vi "Close.vi"(8 "error in (no error)":errorcluster, 11 "Data.TDMS in":refnum<class "Data.PG.lvclass">) -> (0 "error out":errorcluster, 3 "Data.TDMS out":refnum<class "Data.PG.lvclass">)   [LabVIEW 2020, in "Data.PG.lvclass"]
uses:
  Data.PG.lvclass
  <vilib>/JDP Science/PostgreSQL Library/Connection/PQ Connection.lvclass
  Data.PG.lvclass/Data.PG.ctl
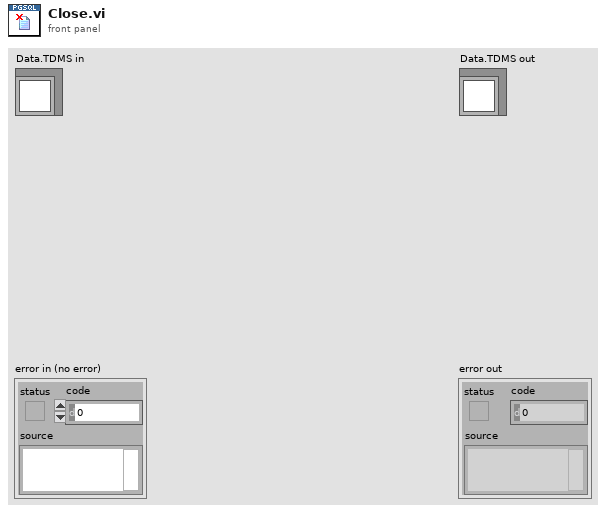
[diagram p1: front panel]
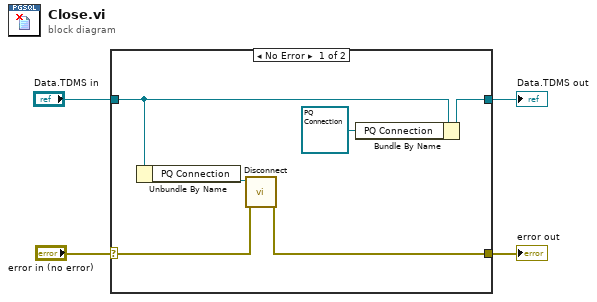
[diagram p0: block diagram]
diagram:
  n1 = case shown="No Error" "error in (no error)" {
    selector: "error in (no error)" -> [w8 w12]
    tunnel: [w9 w11] -> w4
    tunnel: "Data.TDMS in" -> [w6 w11]
    tunnel: [w7 w12] -> w1
    frame No Error {
      n2 = Unbundle By Name(w6) -> ("PQ Connection"=w5:refnum<class "PQ Connection.lvclass">)
      n3 = call-dynamic "Disconnect.vi"("error in (no error)"=w8, "PQ Connection in"=w5) -> ("error out"=w7:errorcluster)  [unwired: 9 in]
      n4 = Bundle By Name(cluster=w6, "PQ Connection"=refnum<class "PQ Connection.lvclass"> refnum) -> (w9:refnum<class "Data.PG.lvclass">)
    }
    frame Error {
    }
  }
  "error out" <- w1
  "Data.TDMS out" <- w4
